vi "fake tool add.vi"(10 "y":dbl, 11 "x":dbl) -> (3 "x+y":dbl)   [LabVIEW 2020, in "MCP Server tests.lvlib"]
doc: "This is a fake tool to test the MCP server toolkit. It adds two numbers and returns the result."
uses:
  MCP Server tests.lvlib
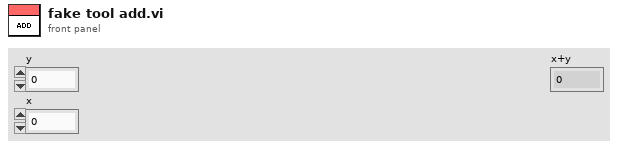
[diagram p1: front panel]
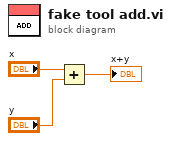
[diagram p0: block diagram]
diagram:
  n1 = Add(x="x", y="y") -> (x+y=→"x+y":dbl)
